vi "initialise.vi"(8 "error in (no error)":errorcluster, 10 "HWList":string[](array[string]), 11 "AtomChipHWC in":refnum<class "AtomChipHWC.lvclass">) -> (0 "error out":errorcluster, 3 "AtomChipHWC out":refnum<class "AtomChipHWC.lvclass">)   [LabVIEW 2011, in "Hardware.lvlib" / "HWControllers.lvlib" / "AtomChipHWC.lvclass"]
doc: "Initialise the devices in the list"
uses:
  AtomChipHWC.lvclass
  HWController.lvclass
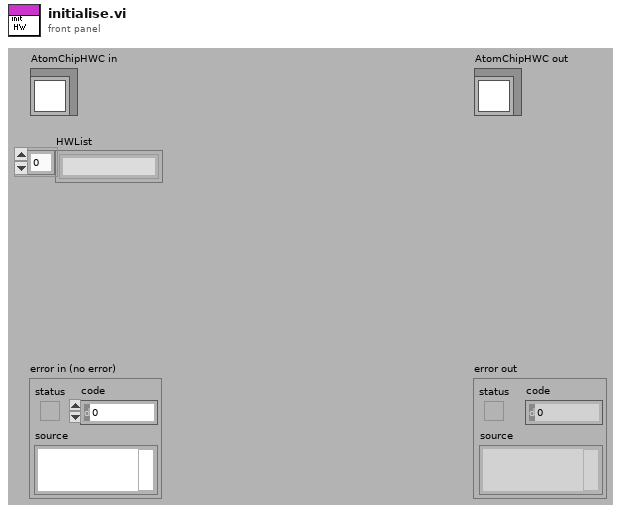
[diagram p1: front panel]
types:
  T1 = enum16{"Ready", "Compiling", "Configured", "Running", "Stopping", "Unresolved Error"}
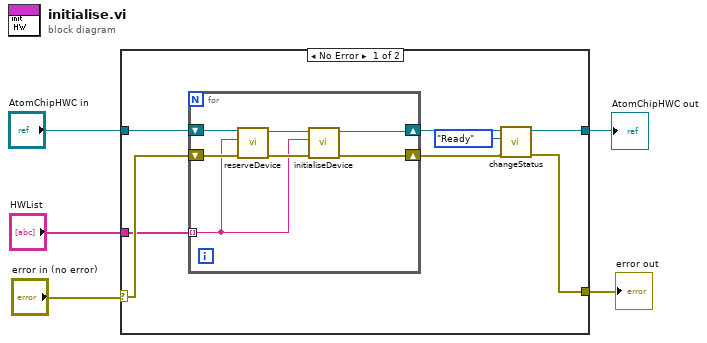
[diagram p0: block diagram]
diagram:
  n1 = case shown="No Error" "error in (no error)" {
    selector: "error in (no error)" -> [w12 w21]
    tunnel: "AtomChipHWC in" -> [w13 w22]
    tunnel: [w10 w22] -> w3
    tunnel: [w8 w21] -> w2
    tunnel: "HWList" -> [w11 _]
    frame No Error {
      n2 = for {
        shift-right: [w15] -> w7
        shift-left: w13 -> [w20]
        tunnel: w11 -> [w16] mode=indexing
        shift-right: [w14] -> w9
        shift-left: w12 -> [w19]
        n3 = call "reserveDevice.vi"("error in (no error)"=w19, "deviceName"=w16, "HWController in"=w20) -> ("error out"=w18:errorcluster, "HWController out"=w17:refnum<class "AtomChipHWC.lvclass">)  [unwired: 7 in]
        n4 = call "initialiseDevice.vi"("error in (no error)"=w18, "deviceName"=w16, "AtomChipHWC in"=w17) -> ("error out"=w14:errorcluster, "AtomChipHWC out"=w15:refnum<class "AtomChipHWC.lvclass">)  [unwired: 7 in]
      }
      n5 = call "changeStatus.vi"("error in (no error)"=w9, "status"=T1."Ready", "HWController in"=w7) -> ("error out"=w8:errorcluster, "HWController out"=w10:refnum<class "AtomChipHWC.lvclass">)  [unwired: 7 in]
    }
    frame Error {
    }
  }
  "error out" <- w2
  "AtomChipHWC out" <- w3
